vi "Toolbox 2 way communication.vi"() -> ()   [LabVIEW 2011]
uses:
  <vilib>/LabVIEW Interface for Arduino/Type Defs/Connection Type.ctl
  <vilib>/LabVIEW Interface for Arduino/Type Defs/Board Type.ctl
  <vilib>/LabVIEW Interface for Arduino/LabVIEW Interface for Arduino.lvlib
panel:
  in  "Tab Control":enum32{"Settings", "Page 2"}(tab)
  in  "VISA resource name":refnum<visa-resource-name>
  in  "Stop Button":bool
  in  "Baud Rate":u32
  in  "Connection Type":T1
  in  "Board Type":T2
  out "Error Out":errorcluster
  out "Waveform Chart":dbl(graph)
  out "Boolean":bool
  out "X":dbl(slide) scale=0.0..5.0
  out "Y":dbl(slide) scale=0.0..5.0
  in  "Numeric Control 2":u8(knob) scale=0.0..10.0
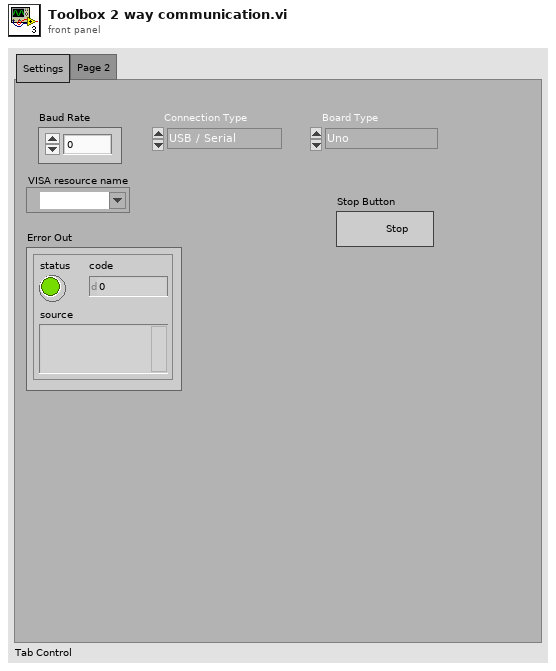
[diagram p1: front panel]
types:
  T1 = typedef "LabVIEW Interface for Arduino.lvlib/Connection Type.ctl" = enum8{"USB / Serial", "XBEE", "BlueSmirf (Bluetooth)"}
  T2 = typedef "LabVIEW Interface for Arduino.lvlib/Board Type.ctl" = enum16{"Uno", "Dimuelanove w/Atmega 328", "Mega 2560"}
  T3 = typedef "LabVIEW Interface for Arduino.lvlib/Arduino Resource.ctl" = cluster{"VISA resource":refnum<visa-resource-name>, "Board Type":T2, "Connection Type":enum8{"USB / Serial"}, "Bytes Per Packet (15)":u8}
  T4 = cluster{"Horizontal Axis Pin":dbl, "Vertical Axis Pin":dbl, "Select Pin":dbl}
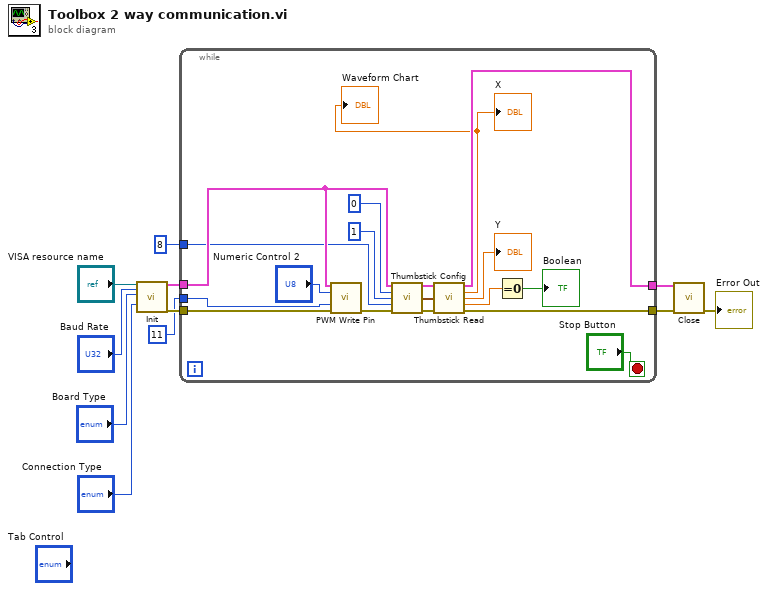
[diagram p0: block diagram]
diagram:
  n1 = call <vilib>:"Init.vi"("VISA resource"="VISA resource name", "Baud Rate (115200)"="Baud Rate", "Board Type (Uno)"="Board Type", "Connection Type (USB/Serial)"="Connection Type") -> ("Arduino Resource"=w8:T3, "error out"=w7:errorcluster)  [unwired: 14 in]
  n2 = while {
    tunnel: w8 -> [w26]
    tunnel: w7 -> [w28]
    tunnel: [w19] -> w5
    tunnel: [w18] -> w4
    tunnel: 11 -> [w17]
    tunnel: 8 -> [w16]
    stop <- "Stop Button" stop-if-true
    n3 = call <vilib>:"PWM Write Pin.vi"("Arduino Resource"=w26, "Duty Cycle (0 - 255)"="Numeric Control 2", "PWM Pin (3)"=w17, "error in"=w28) -> ("error out"=w20:errorcluster)  [unwired: 10 in, 1 out]
    n4 = call <vilib>:"Thumbstick Config.vi"("Arduino Resource"=w26, "Horizontal Axis AI Pin"=0, "Vertical Axis AI Pin"=1, "Select DI Pin"=w16, "error in"=w20) -> ("Arduino Resource"=w22:T3, "Thumbstick Data"=w23:T4, "error out"=w21:errorcluster)  [unwired: 8 in]
    n5 = call <vilib>:"Thumbstick Read.vi"("Arduino Resource"=w22, "Thumbstick Data"=w23, "error in"=w21) -> ("Arduino Resource"=w19:T3, "Horizontal Axis"=→"X" →"Waveform Chart":dbl, "Vertical Axis"=→"Y":dbl, "Select (Active Low)"=w15:dbl, "error out"=w18:errorcluster)  [unwired: 8 in]
    n6 = Equal To 0?(x=w15) -> (x = 0?=→"Boolean":bool)
  }
  n7 = call <vilib>:"Close.vi"("Arduino Resource"=w5, "error in"=w4) -> ("error out"=→"Error Out":errorcluster)  [unwired: 13 in]
